vi "HGCalSensorTestingPanel4.vi"() -> ()   [LabVIEW 2015]
uses:
  <vilib>/Utility/file.llb/Read Delimited Spreadsheet (DBL).vi
  <vilib>/Utility/file.llb/Read Delimited Spreadsheet (I64).vi
  <vilib>/Utility/file.llb/Write Delimited Spreadsheet (string).vi
panel:
  out "XY Graph 3":cluster{"Y":dbl[], "Y":dbl[]}[](graph)
  out "HP count":u32
  in  "HP read count":u32
  in  "HP VISA":refnum<visa-resource-name>
  out "K237 count":u32
  in  "K237 VISA":refnum<visa-resource-name>
  out "XY Graph 2":cluster{"Y":dbl[], "Y":dbl[]}[](graph)
  out "return count 5":u32
  in  "write buffer 2":string
  out "return count 4":u32
  in  "QT VISA":refnum<visa-resource-name>
  in  "write buffer":string
  out "return count 3":u32
  in  "byte count 2":u32
  out "XY Graph":cluster{"Y":dbl[], "Y":dbl[]}[](graph)
  out "return count":u32
  in  "K706 VISA":refnum<visa-resource-name>
  in  "Measurement Data":string[][](table)
  in  "OK Button":bool
  in  "Delay (s):":dbl
  in  "Channel:":dbl
  in  "Voltage (V):":dbl
  out "Channel:":dbl format="%#3_6g"
  out "mV(nA)":dbl
  out "pF":dbl
  out "V":dbl
  out "nA":dbl
  # "C"
  # "A"
  # "V"
  # "1M"
  # "1M"
  # "Single Measurement"
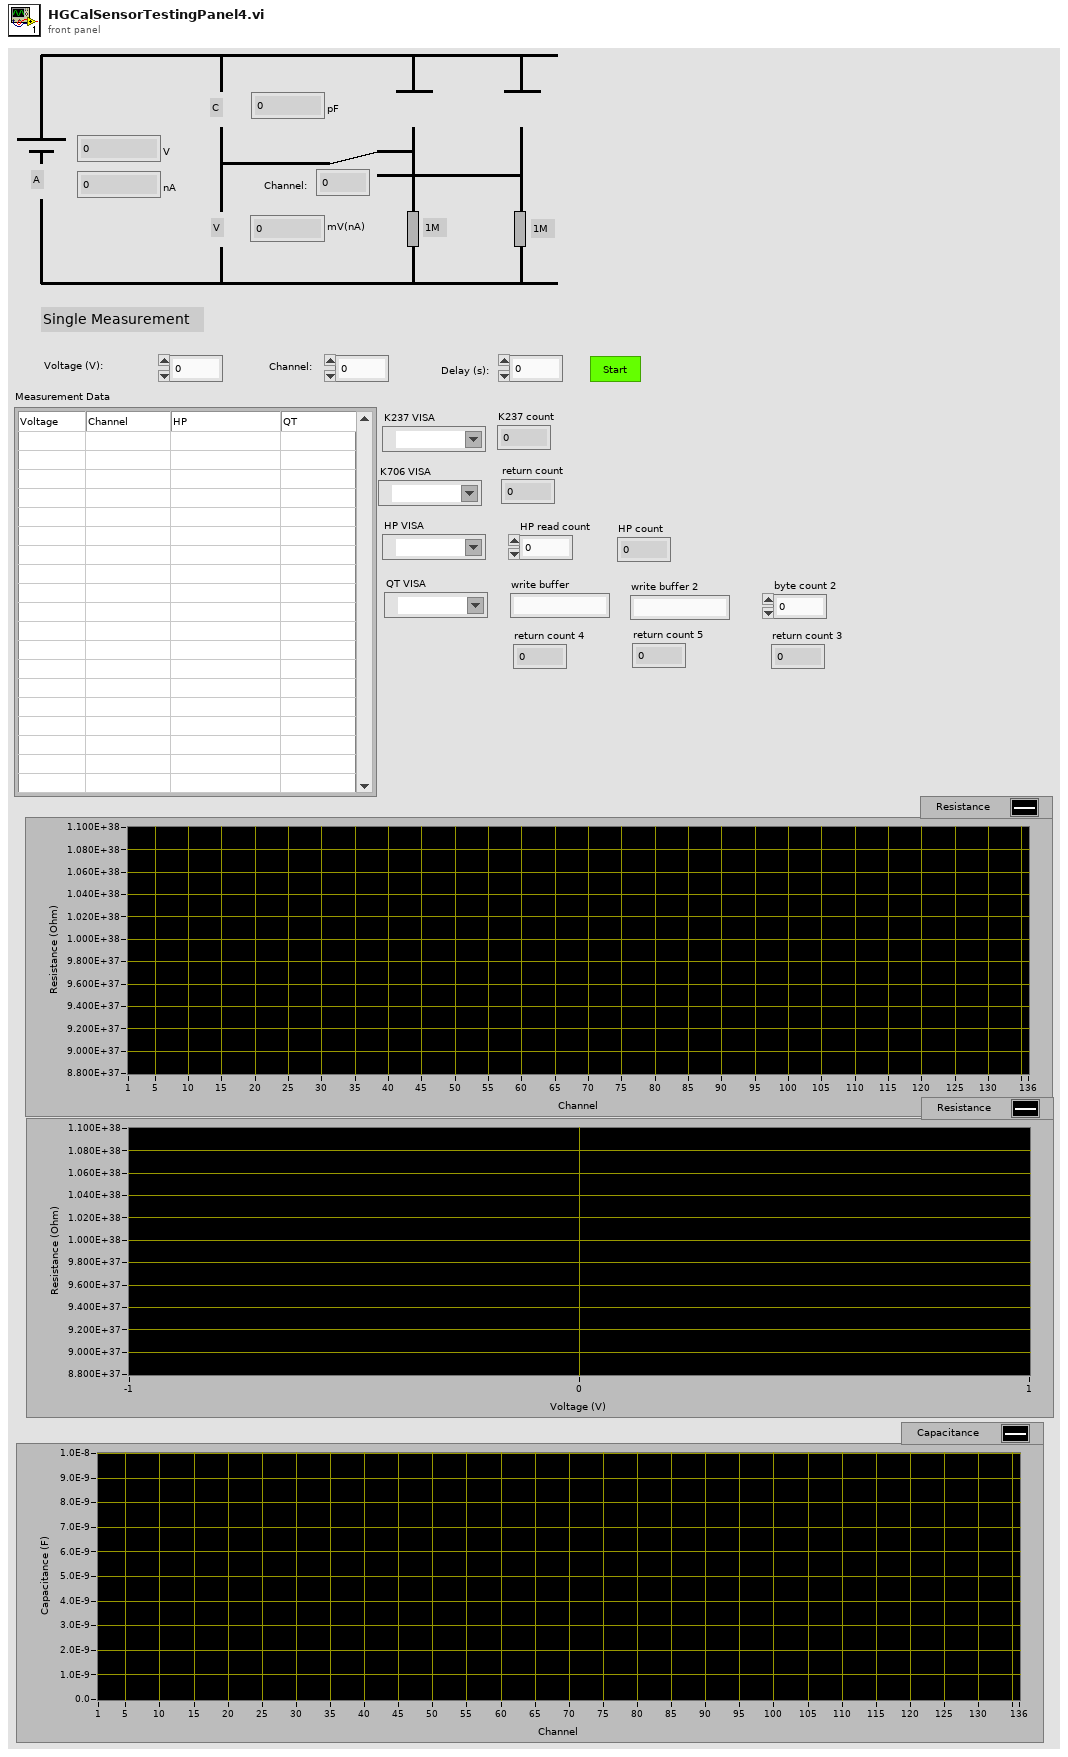
[diagram p1: front panel]
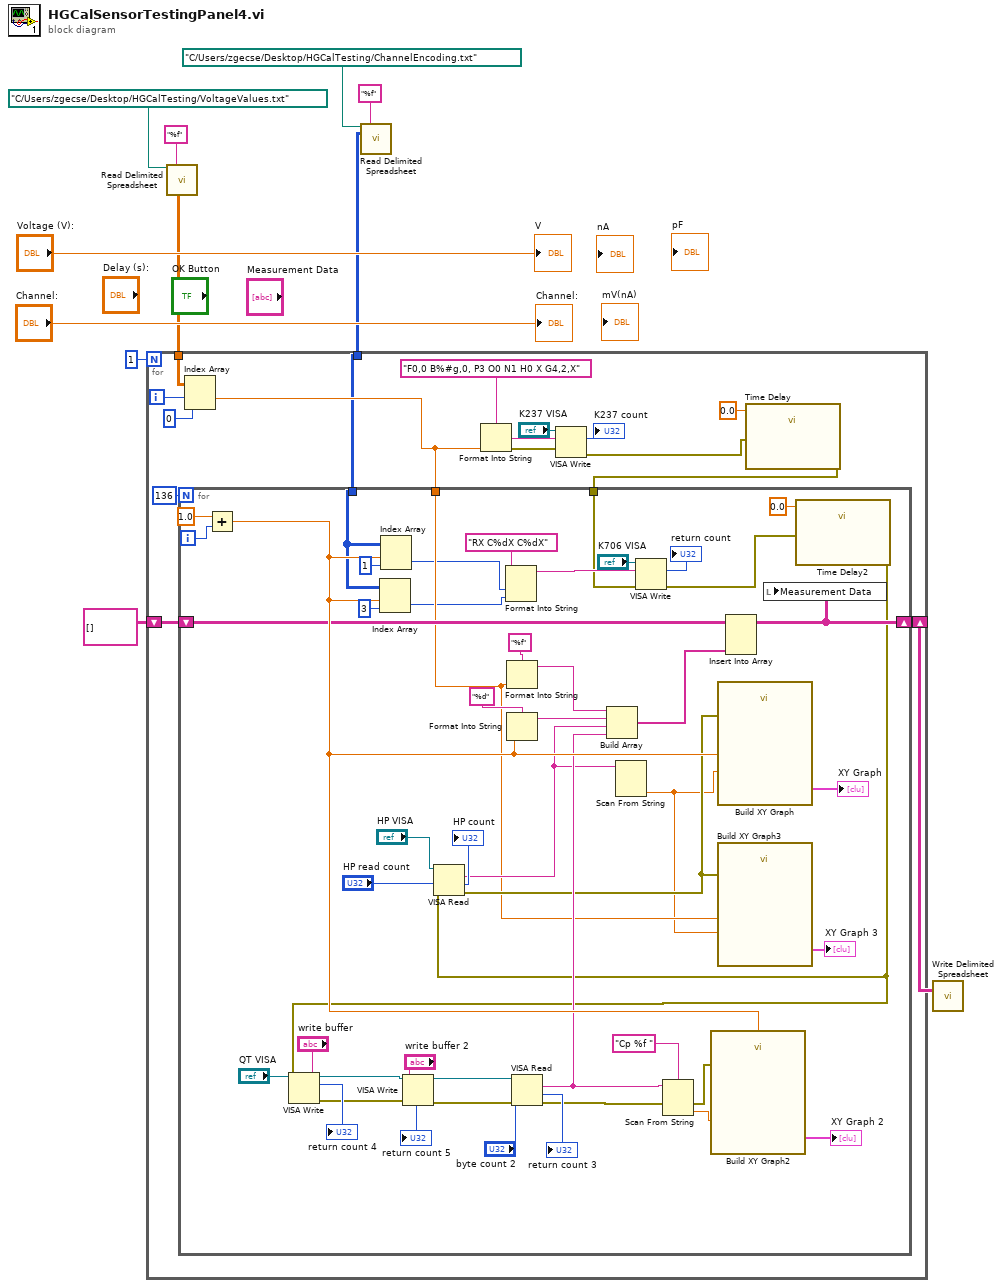
[diagram p0: block diagram]
diagram:
  n1 = call-poly <vilib>:"Read Delimited Spreadsheet.vi"("file path (dialog if empty)"=path "C:/Users/zgecse/Desktop/HGCalTesting/VoltageValues.txt", "format (%.3f)"="%f") -> ("all rows"=w4:dbl[][])  [unwired: 8 in, 5 out]
  n2 = call-poly <vilib>:"Read Delimited Spreadsheet.vi"("file path (dialog if empty)"=path "C:/Users/zgecse/Desktop/HGCalTesting/ChannelEncoding.txt", "format (%d)"="%f" ("format (%.3f)")) -> ("all rows"=w1:i64[][])  [unwired: 8 in, 5 out]
  n3 = for {
    N: 1 -> [_]
    shift-right: [w25] -> w8
    shift-left: string[][] [] -> [w27]
    tunnel: w4 -> [w17]
    tunnel: w1 -> [w12]
    i -> [w19]
    n4 = Index Array(array=w17, index (row)=w19, index (col)=0 ("disabled index (col)")) -> (element=w18:dbl)
    n5 = Format Into String(format string="F0,0 B%#g,0, P3 O0 N1 H0 X G4,2,X" ("F0,0X B%f,0,X L%f,0X P3X O0X"), w18) -> (resulting string=w20:string, error out=w21:errorcluster)  [unwired: 2 in]
    n6 = VISA Write(VISA resource name="K237 VISA", write buffer=w20, error in (no error)=w21) -> (return count=→"K237 count":u32, error out=w15:errorcluster)  [unwired: 1 out]
    n7 = call "Time Delay"("error in (no error)"=w15, "Delay Time (s)"=0.0) -> ("error out"=w14:errorcluster)  [unwired: 9 in]
    n8 = for {
      N: 136 -> [_]
      shift-right: [w44] -> w25
      shift-left: w27 -> [w45]
      tunnel: w14 -> [w46]
      tunnel: w18 -> [w35]
      tunnel: w12 -> [w32]
      i -> [w71]
      n9 = Add(x=1.0, y=w71) -> (x+y=w52:dbl)
      n10 = Index Array(array=w32, index (row)=w52, index (col)=3 ("disabled index (col)")) -> (element=w28:i64)
      n11 = Index Array(array=w32, index (row)=w52, index (col)=1 ("disabled index (col)")) -> (element=w29:i64)
      n12 = Format Into String(format string="RX C%dX C%dX", w29, w28) -> (resulting string=w68:string)  [unwired: 2 in, 1 out]
      n13 = Format Into String(format string="%f", w35) -> (resulting string=w76:string)  [unwired: 2 in, 1 out]
      n14 = Format Into String(format string="%d", w52) -> (resulting string=w66:string)  [unwired: 2 in, 1 out]
      n15 = VISA Write(VISA resource name="K706 VISA", write buffer=w68, error in (no error)=w46) -> (return count=→"return count":u32, error out=w42:errorcluster)  [unwired: 1 out]
      n16 = call "Time Delay2"("error in (no error)"=w42, "Delay Time (s)"=0.0) -> ("error out"=w37:errorcluster)  [unwired: 9 in]
      n17 = VISA Write(VISA resource name="QT VISA", write buffer="write buffer", error in (no error)=w37) -> (VISA resource name out=w55:refnum<visa-resource-name>, return count=→"return count 4":u32, error out=w57:errorcluster)
      n18 = VISA Write(VISA resource name=w55, write buffer="write buffer 2", error in (no error)=w57) -> (VISA resource name out=w54:refnum<visa-resource-name>, return count=→"return count 5":u32, error out=w56:errorcluster)
      n19 = VISA Read(VISA resource name="HP VISA", byte count="HP read count", error in (no error)=w37) -> (read buffer=w38:string, return count=→"HP count":u32, error out=w36:errorcluster)  [unwired: 1 out]
      n20 = VISA Read(VISA resource name=w54, byte count="byte count 2", error in (no error)=w56) -> (read buffer=w50:string, return count=→"return count 3":u32, error out=w49:errorcluster)  [unwired: 1 out]
      n21 = Build Array(w76, w66, w38, w50) -> (w75:string[])
      n22 = Scan From String(input string=w38) -> (output 1=w34:dbl)  [unwired: 4 in, 3 out]
      n23 = Scan From String(format string="Cp %f ", input string=w50, error in=w49) -> (error out=w48:errorcluster, output 1=w51:dbl)  [unwired: 2 in, 2 out]
      n24 = call "Build XY Graph2"("error in (no error)"=w48, "Y Input"=w51, "X Input"=w52) -> ("XY Graph"=→"XY Graph 2":cluster{"X":dbl[], "Y":dbl[]}[])  [unwired: 7 in, 1 out]
      n25 = call "Build XY Graph"("error in (no error)"=w36, "Y Input"=w34, "X Input"=w52) -> ("XY Graph"=→"XY Graph":cluster{"X":dbl[], "Y":dbl[]}[])  [unwired: 7 in, 1 out]
      n26 = call "Build XY Graph3"("error in (no error)"=w36, "Y Input"=w34, "X Input"=w35) -> ("XY Graph"=→"XY Graph 3":cluster{"X":dbl[], "Y":dbl[]}[])  [unwired: 7 in, 1 out]
      n27 = Insert Into Array(array=w45, new element=w75) -> (w44:string[][])  [unwired: 2 in]
      n28 = local write "Measurement Data"(w44) -> ()
    }
  }
  n29 = call-poly <vilib>:"Write Delimited Spreadsheet.vi"("2D data"=w8) -> ()  [unwired: 13 in, 2 out]
  "V" <- "Voltage (V):"
  "Channel:" <- "Channel:"
